vi "front panel to new coordinates.vi"(1 "new top":i16=24, 7 "path":path, 11 "error in (no error)":errorcluster, 12 "new left":i16=4) -> (15 "error out":errorcluster)   [LabVIEW 2016]
doc: "this vi uses VI reference poperties to move the front panel to the upper left corner of the screen.\n\nPaul K Dixon\nPhysics 350\nCSUSB Physics"
uses:
  <vilib>/Utility/miscctls.llb/LVRectTypeDef.ctl
panel:
  out "Window Bounds Out":T1
  out "Window Bounds In":T1
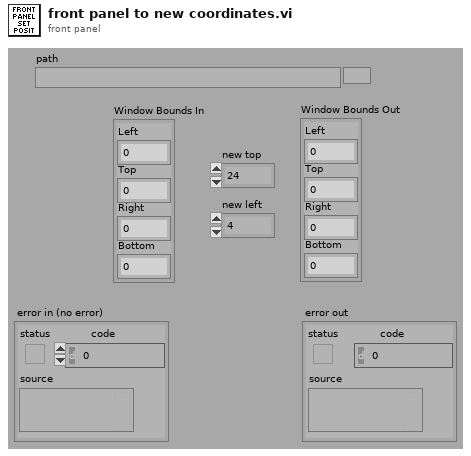
[diagram p1: front panel]
types:
  T1 = typedef "LVRectTypeDef.ctl" = cluster{"Left":i16, "Top":i16, "Right":i16, "Bottom":i16}
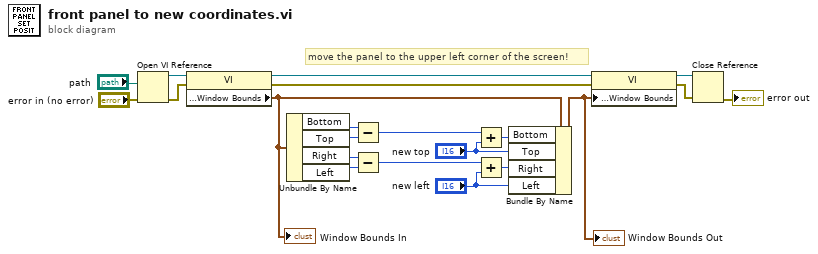
[diagram p0: block diagram]
diagram:
  # "move the panel to the upper left corner of the screen!"
  n1 = Open VI Reference(vi path="path", error in (no error)="error in (no error)") -> (vi reference=w8:refnum<vi>, error out=w17:errorcluster)  [unwired: 4 out]
  n2 = property class="VI"(reference=w8, error in=w17) -> (reference out=w9:refnum<vi>, error out=w18:errorcluster, "Front Panel Window:Window Bounds"=w15:T1)
  "Window Bounds In" <- w15
  n3 = Unbundle By Name(w15) -> ("Bottom"=w10:i16, "Top"=w11:i16, "Right"=w12:i16, "Left"=w13:i16)
  n4 = Subtract(x=w10, y=w11) -> (x-y=w5:i16)
  n5 = Subtract(x=w12, y=w13) -> (x-y=w1:i16)
  n6 = Add(x=w5, y="new top") -> (x+y=w4:i16)
  n7 = Add(x=w1, y="new left") -> (x+y=w2:i16)
  n8 = Bundle By Name(cluster=w15, "Bottom"=w4, "Top"="new top", "Right"=w2, "Left"="new left") -> (w7:T1)
  "Window Bounds Out" <- w7
  n9 = property class="VI"(reference=w9, error in=w18, "Front Panel Window:Window Bounds"=w7) -> (reference out=w16:refnum<vi>, error out=w19:errorcluster)
  n10 = Close Reference(reference=w16, error in (no error)=w19) -> (error out=→"error out":errorcluster)
